vi "Update Queue Nested.vi"(10 "Queue Nested":map{string, refnum<data-value>}(c390), 11 "Update Queue Nested in":refnum<class "Update Queue Nested.lvclass">) -> (3 "Update Queue Nested out":refnum<class "Update Queue Nested.lvclass">)   [LabVIEW 2021, in "Update Queue Nested.lvlib" / "Update Queue Nested.lvclass"]
uses:
  Update Queue Nested.lvclass
  Msg/Msg.lvclass
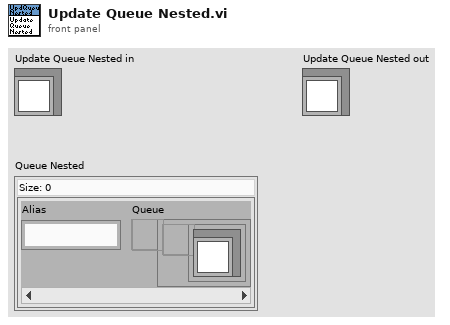
[diagram p1: front panel]
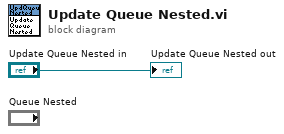
[diagram p0: block diagram]
diagram:
  "Update Queue Nested out" <- "Update Queue Nested in"
